vi "testMaxFileSize (text file - not exceeded).vi"(8 "error in (no error)":errorcluster, 11 "TestCase in":refnum<class "Test Max File Size.lvclass">) -> (0 "error out":errorcluster, 3 "TestCase out":refnum<class "Test Max File Size.lvclass">)   [LabVIEW 2019, in "Test Max File Size.lvclass"]
uses:
  Test Max File Size.lvclass
  C:/Program Files/National Instruments/LabVIEW 2024/vi.lib/Astemes/LUnit/Test Case.lvclass
  Log Sinks/Text File/Text File.lvclass
  C:/Development/Open Source/tsc-event-logger/Log Sinks/Log Sinks.lvclass
  Log/Event Level.ctl
  Log/Log.lvclass/Log.ctl
  Log Sinks/Text File/Text File.lvclass/Text File.ctl
  <vilib>/Astemes/LUnit/Test Case.lvclass/Test Case.ctl
  4449ac42-d49d-42f3-b37d-ed8064ff559b.vi
  837c3ff2-8343-4b8b-8377-434b4b4b8461.vi
  <vilib>/Astemes/LUnit/Core/LUnit Test Case/Private/Append Pass Result.vi
  <vilib>/Astemes/LUnit/Core/LUnit Test Case/Private/Append Fail Result.vi
  837c3ff2-8343-4b8b-8377-434b4b4b8461.vi/9c5d11cd-9439-4240-a1ee-d9baace9c924.vi
  <vilib>/Astemes/LUnit/Core/LUnit Test Case/Private/Run In UI.vi
  <vilib>/Utility/error.llb/Clear Errors.vi
  Log Sinks/Send Log Packet.vi
  TSC Event Logger.lvlib
  Log/Log.lvclass
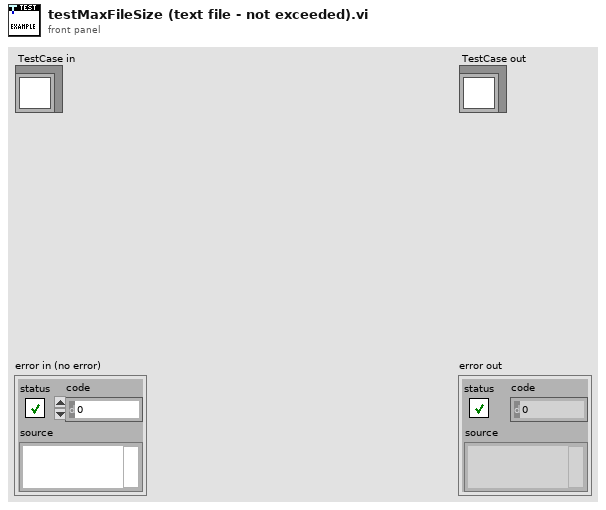
[diagram p1: front panel]
types:
  T1 = typedef "TSC Event Logger.lvlib/Event Level.ctl" = enum16{"OFF", "TRACE", "DEBUG", "INFO", "WARN", "ERROR", "FATAL"}
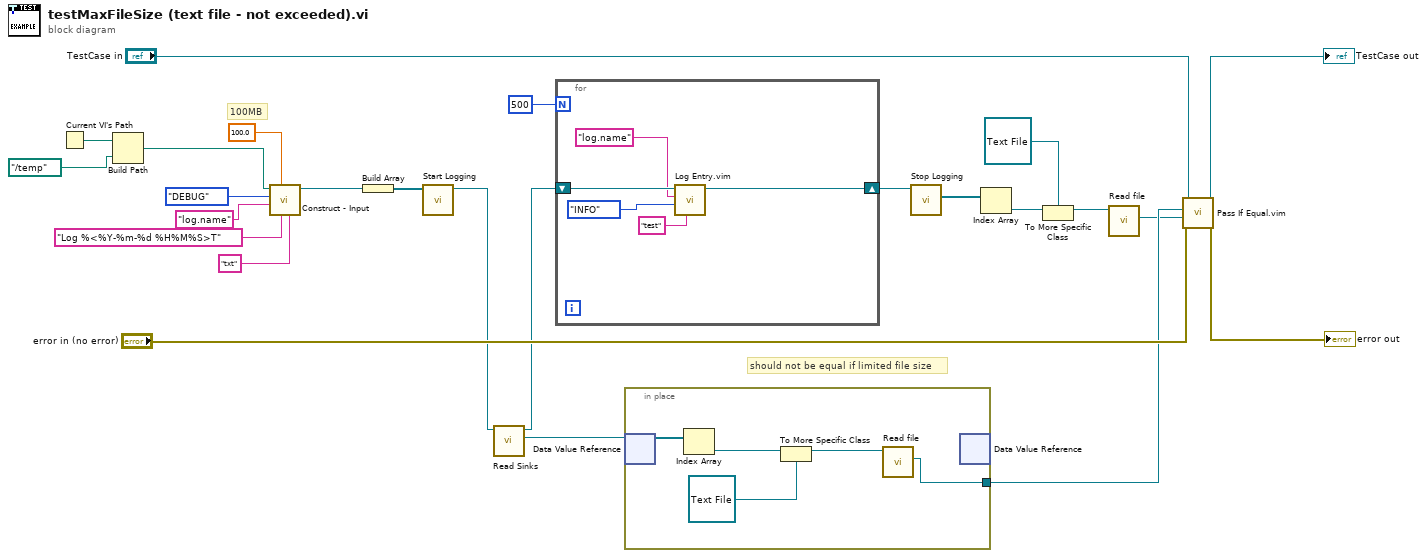
[diagram p0: block diagram]
diagram:
  # "100MB"
  # "should not be equal if limited file size"
  n1 = Current VI's Path() -> (path=w9:path)
  n2 = Build Path(base path=w9, name or relative path=path "../temp") -> (appended path=w11:path)
  n3 = call "Construct - Input.vi"("extension"="txt", "file name format"="Log %<%Y-%m-%d %H%M%S>T", "Max File Size (MB)"=100.0, "Name"="log.name", "Level"=Event_Level."DEBUG", "log location"=w11) -> ("Text File"=w4:refnum<class "Text File.lvclass">)  [unwired: 4 in, 1 out]
  n4 = Build Array(w4) -> (w3:refnum<class "Text File.lvclass">[])
  n5 = call "Start Logging.vi"("Sinks"=w3) -> ("Logger"=w1:refnum<class "Log.lvclass">)  [unwired: 9 in, 1 out]
  n6 = call "Read Sinks.vi"("Log in"=w1) -> ("Sink DVR Array"=w21:refnum<data-value>, "Log out"=w16:refnum<class "Log.lvclass">)  [unwired: 9 in]
  n7 = for {
    N: 500 -> [_]
    shift-right: [w28] -> w17
    shift-left: w16 -> [w29]
    n8 = call "Log Entry.vim"("Message"="test", "Level"=Event_Level."INFO", "Logger"="log.name", "Log in"=w29) -> ("Log out"=w28:refnum<class "Log.lvclass">)  [unwired: 6 in, 1 out]
  }
  n9 = in-place {
    in-place-border: [w31] -> w20
    n10 = in-place-dvr #1(w21) -> (w35:refnum<class "Log Sinks.lvclass">[])  [unwired: 1 out]
    n11 = Index Array(array=w35) -> (element=w34:refnum<class "Log Sinks.lvclass">)  [unwired: 1 in]
    n12 = To More Specific Class(target class=refnum<class "Text File.lvclass"> refnum ("TSC Event Logger.lvlib:Text File.lvclass"), reference=w34) -> (specific class reference=w33:refnum<class "Text File.lvclass">)  [unwired: 1 in, 1 out]
    n13 = call "Read file.vi"("Text File in"=w33) -> ("file"=w31:refnum<file>)  [unwired: 9 in, 1 out]
    n14 = in-place-dvr #1() -> ()  [unwired: 1 in, 2 out]
  }
  n15 = call "Stop Logging.vi"("Logger"=w17) -> ("sinks"=w12:refnum<class "Log Sinks.lvclass">[])  [unwired: 9 in, 1 out]
  n16 = Index Array(array=w12) -> (element=w15:refnum<class "Log Sinks.lvclass">)  [unwired: 1 in]
  n17 = To More Specific Class(target class=refnum<class "Text File.lvclass"> refnum ("TSC Event Logger.lvlib:Text File.lvclass"), reference=w15) -> (specific class reference=w14:refnum<class "Text File.lvclass">)  [unwired: 1 in, 1 out]
  n18 = call "Read file.vi"("Text File in"=w14) -> ("file"=w18:refnum<file>)  [unwired: 9 in, 1 out]
  n19 = call "Pass If Equal.vim"("error in (no error)"="error in (no error)", "Actual"=w18, "Expected"=w20, "LUnit Test Case In"="TestCase in") -> ("error out"=→"error out":errorcluster, "LUnit Test Case Out"=→"TestCase out":refnum<class "Test Max File Size.lvclass">)  [unwired: 6 in]
